vi "Split_Data.vi"(0 "Format_String (%s)":string="%s", 1 "Delimiter":string="\n", 5 "Data_In":string, 11 "Error_In":errorcluster) -> (4 "Split_Data_Out":string[](array[string]), 15 "Error_Out":errorcluster)   [LabVIEW 2023, in "File_Handler_Library.lvlib"]
doc: "This VI Splits string data and forms array"
uses:
  File_Handler_Library.lvlib
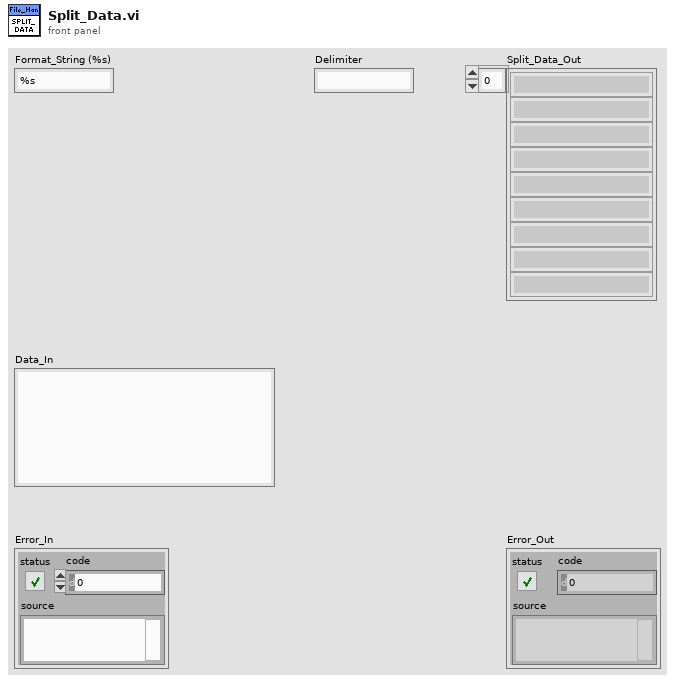
[diagram p1: front panel]
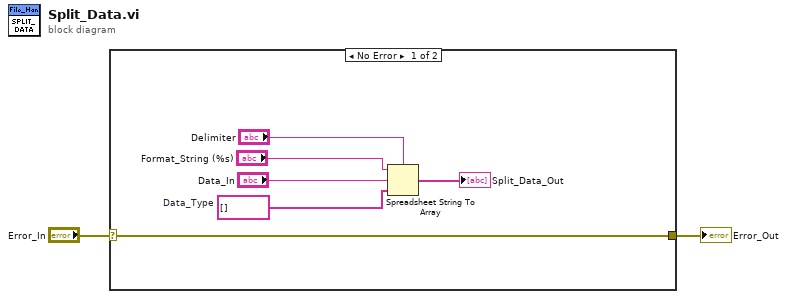
[diagram p0: block diagram]
diagram:
  n1 = case shown="No Error" "Error_In" {
    selector: "Error_In" -> [w3 w9]
    tunnel: [w3 w9] -> w1
    frame No Error {
      w5 = string[] []  # Data_Type
      n2 = Spreadsheet String To Array(delimiter (Tab)="Delimiter", format string="Format_String (%s)", spreadsheet string="Data_In", array type (2D Dbl)=w5) -> (array=→"Split_Data_Out":string[])
    }
    frame Error {
    }
  }
  "Error_Out" <- w1
